vi "Build ADU_ASCII.vi"(8 "error in (no error)":errorcluster, 10 "Slave Address":u8) -> (0 "error out":errorcluster, 3 "MB_ADU_ASCII out":refnum<class "MB_ADU_ASCII.lvclass">)   [LabVIEW 2016, in "MB Master.lvlib" / "MB_ADU_ASCII.lvclass"]
doc: "Builds an ADU for Modbus ASCII mode."
uses:
  MB_ADU_ASCII.lvclass
  C:/Users/illogicdev/Desktop/IGUS/20190906-1xdryveD1+LABview+ModbusTCP(Gateway)/IgusPositioningSystem Folder/Modules/Libraries/Modbus-Master/MB_ADU/MB_ADU.lvclass
  MB_ADU/MB_ADU.lvclass/MB_ADU.ctl
  MB_ADU/MB_ADU.lvclass
panel:
  in  "MB_ADU_ASCII in":refnum<class "MB_ADU_ASCII.lvclass">
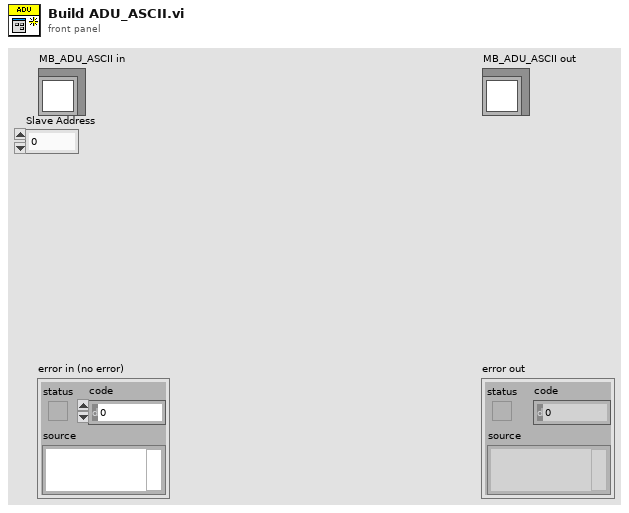
[diagram p1: front panel]
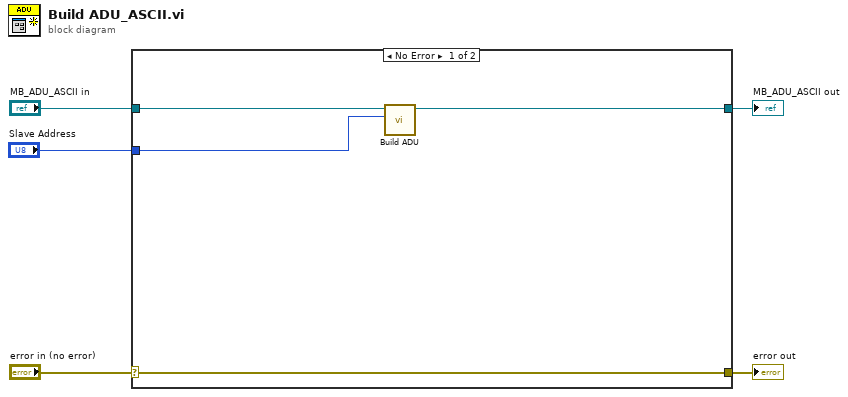
[diagram p0: block diagram]
diagram:
  n1 = case shown="No Error" "error in (no error)" {
    selector: "error in (no error)" -> [w9 w11]
    tunnel: [w9 w11] -> w4
    tunnel: [w7 w10] -> w2
    tunnel: "MB_ADU_ASCII in" -> [w8 w10]
    tunnel: "Slave Address" -> [w6 _]
    frame No Error {
      n2 = call "Build ADU.vi"("Slave ID"=w6, "MB_ADU in"=w8) -> ("MB_ADU out"=w7:refnum<class "MB_ADU_ASCII.lvclass">)  [unwired: 8 in, 1 out]
    }
    frame Error {
    }
  }
  "error out" <- w4
  "MB_ADU_ASCII out" <- w2
